vi "DN4_Counter_ReadPulseWidth_Ex.vi"(2 "error in (no error)":errorcluster, 3 "Task ID":u32) -> (0 "error out":errorcluster, 1 "pulse width":cluster{"high period":dbl, "low period":dbl}[](array[cluster]))   [LabVIEW 2009]
uses:
  Windows/System32/AdvLvDaq.dll
panel:
  in  "PulseWidth":cluster{"high period":dbl, "low period":dbl}
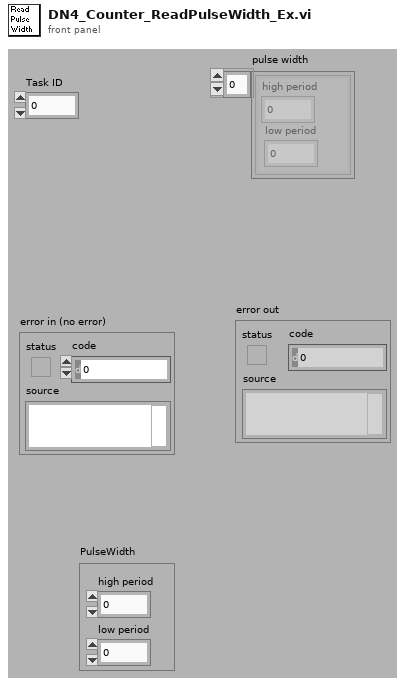
[diagram p1: front panel]
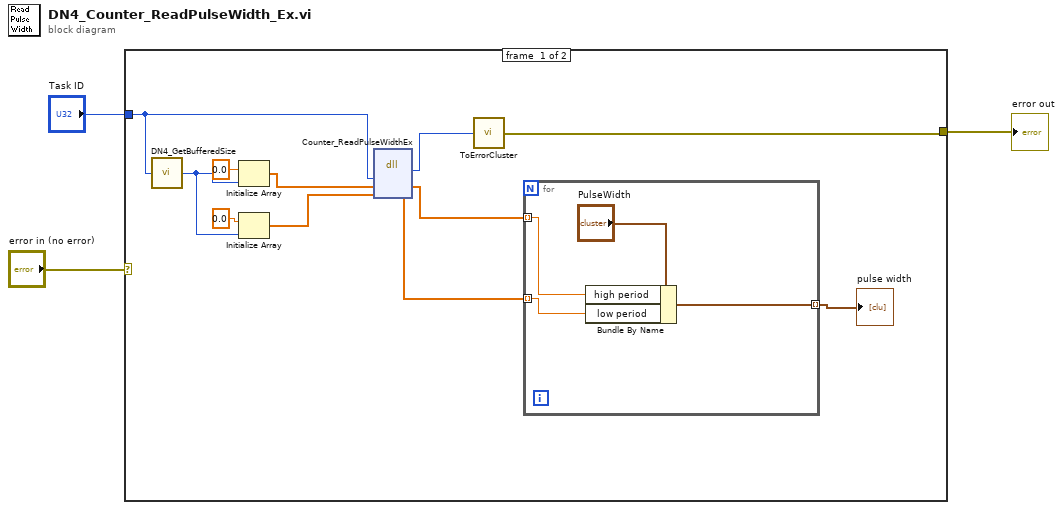
[diagram p0: block diagram]
diagram:
  n1 = case shown="Error" "error in (no error)" {
    selector: "error in (no error)" -> [_ w19]
    tunnel: "Task ID" -> [w14 _]
    tunnel: [w4 w19] -> w1
    frame #0 {
      n2 = call <userlib>:"DN4_GetBufferedSize.vi"("Task ID"=w14) -> ("return type"=w11:i32)
      n3 = Initialize Array(0.0 ("element"), w11) -> (w10:dbl[])
      n4 = Initialize Array(0.0 ("element"), w11) -> (w9:dbl[])
      n5 = dll-call lib="C:/Windows/System32/AdvLvDaq.dll" fn="Counter_ReadPulseWidthEx"("taskId"=w14, "highPeriods"=w10, "lowPeriods"=w9) -> ("return type"=w5:i32, "highPeriods"=w8:dbl[], "lowPeriods"=w7:dbl[])  [unwired: 4 in, 2 out]
      n6 = call <userlib>:"ToErrorCluster.vi"("error code"=w5) -> ("error out"=w4:errorcluster)
      n7 = for {
        tunnel: w8 -> [w17] mode=indexing
        tunnel: w7 -> [w16] mode=indexing
        tunnel: [w15] -> w6 mode=indexing
        n8 = Bundle By Name(cluster="PulseWidth", "high period"=w17, "low period"=w16) -> (w15:cluster{"high period":dbl, "low period":dbl})
      }
      "pulse width" <- w6
    }
    frame #1 {
    }
  }
  "error out" <- w1
